vi "Close.vi"(8 "Error In":errorcluster, 11 "Central Message Handler":refnum<class "Central Message Handler.lvclass">) -> (0 "Error Out":errorcluster)   [LabVIEW 2021, in "Central Message Handler.lvclass"]
uses:
  Central Message Handler.lvclass
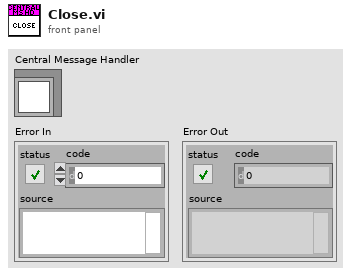
[diagram p1: front panel]
types:
  T1 = typedef "Central Message Handler.lvclass/Data.ctl" = cluster{"Central Message Queue":refnum<queue>, "Processes Queues Map":map{string, refnum<queue>}}
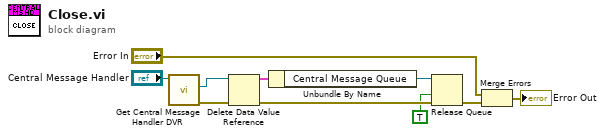
[diagram p0: block diagram]
diagram:
  n1 = call "Get Central Message Handler DVR.vi"("Central Message Handler In"="Central Message Handler") -> ("Error Out"=w8:errorcluster, "DVR"=w9:refnum<data-value>)  [unwired: 8 in, 1 out]
  n2 = Delete Data Value Reference(data value reference=w9, error in=w8) -> (data value=w7:T1, error out=w5:errorcluster)
  n3 = Unbundle By Name(w7) -> ("Central Message Queue"=w6:refnum<queue>)
  n4 = Release Queue(queue=w6, force destroy? (F)=TRUE, error in (no error)=w5) -> (error out=w2:errorcluster)  [unwired: 2 out]
  n5 = Merge Errors("Error In", w2) -> (→"Error Out":errorcluster)
